vi "Simple Spectrometer.vi"() -> ()   [LabVIEW 2013]
uses:
  lightfield-automation-labview/LightField Automation.lvclass
panel:
  in  "ExperimentName":string
  in  "stop":bool
  in  "Center Wavelength":dbl
  in  "Grating":string(combo)
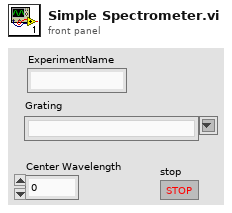
[diagram p1: front panel]
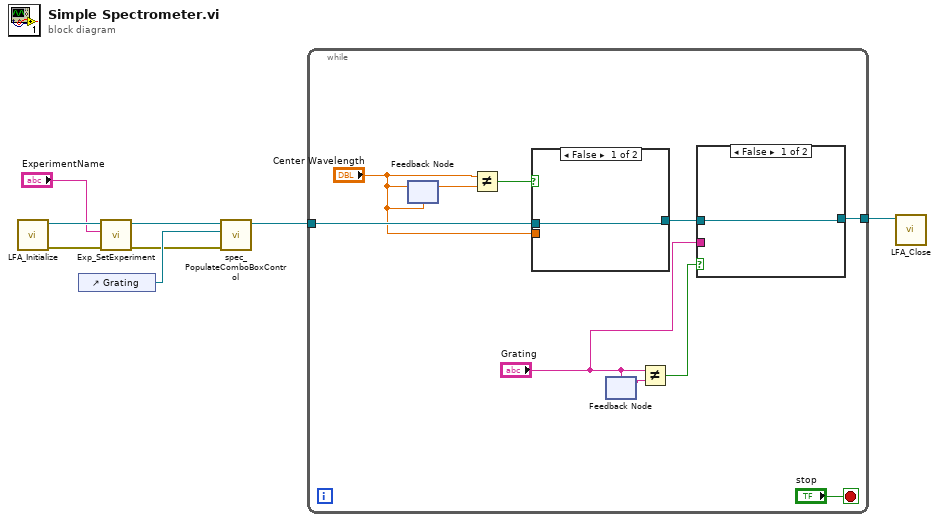
[diagram p0: block diagram]
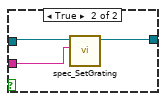
[diagram p2: hidden frame]
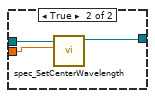
[diagram p3: hidden frame]
diagram:
  n1 = call "LFA_Initialize.vi"() -> ("error out"=w5:errorcluster, "LightField Automation out"=w6:refnum<class "LightField Automation.lvclass">)  [unwired: 10 in]
  n2 = control-ref of="Grating"() -> (w8:refnum<vi>)
  n3 = call "Exp_SetExperiment.vi"("error in (no error)"=w5, "ExperimentName"="ExperimentName", "LightField Automation in"=w6) -> ("error out"=w3:errorcluster, "LightField Automation out"=w2:refnum<class "LightField Automation.lvclass">)  [unwired: 7 in]
  n4 = call "spec_PopulateComboBoxControl.vi"("error in (no error)"=w3, "Combo Box Reference"=w8, "LightField Automation in"=w2) -> ("LightField Automation out"=w7:refnum<class "LightField Automation.lvclass">)  [unwired: 7 in, 1 out]
  n5 = while {
    tunnel: w7 -> [w14]
    tunnel: [w9] -> w1
    stop <- "stop" stop-if-true
    n6 = feedback-in #1("Center Wavelength") -> ()
    n7 = feedback #1("Center Wavelength") -> (w18:dbl)
    n8 = Not Equal?(x="Center Wavelength", y=w18) -> (x != y?=w16:bool)
    n9 = case shown="False" w16 {
      tunnel: w14 -> [w23 w26]
      tunnel: [w23 w25] -> w12
      tunnel: "Center Wavelength" -> [_ w24]
      frame False {
      }
      frame True {
        n10 = call "spec_SetCenterWavelength.vi"("Center Wavelength"=w24, "LightField Automation in"=w26) -> ("LightField Automation out"=w25:refnum<class "LightField Automation.lvclass">)  [unwired: 8 in, 1 out]
      }
    }
    n11 = feedback #2("Grating") -> (w17:string)
    n12 = feedback-in #2("Grating") -> ()
    n13 = Not Equal?(x="Grating", y=w17) -> (x != y?=w15:bool)
    n14 = case shown="False" w15 {
      tunnel: "Grating" -> [_ w22]
      tunnel: w12 -> [w19 w21]
      tunnel: [w19 w20] -> w9
      frame False {
      }
      frame True {
        n15 = call "spec_SetGrating.vi"("GratingSelected"=w22, "LightField Automation in"=w21) -> ("LightField Automation out"=w20:refnum<class "LightField Automation.lvclass">)  [unwired: 8 in, 1 out]
      }
    }
  }
  n16 = call "LFA_Close.vi"("LightField Automation in"=w1) -> ()  [unwired: 9 in, 2 out]
